vi "Latch When Pressed for Time.vi"(4 "Time (ms)":i32, 5 "Input":bool) -> (2 "Latched Output":bool)   [LabVIEW 2014]
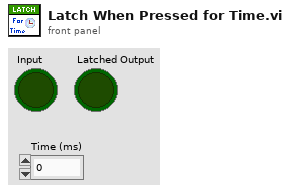
[diagram p1: front panel]
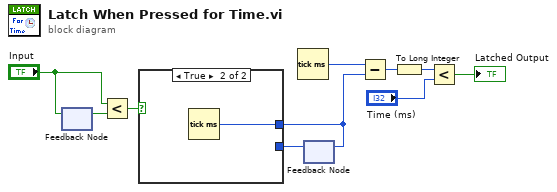
[diagram p0: block diagram]
diagram:
  n1 = feedback-in #1("Input") -> ()
  n2 = feedback #1() -> (w10:bool)  [unwired: 1 in]
  n3 = Less?(x="Input", y=w10) -> (x < y?=w8:bool)
  n4 = Tick Count (ms)() -> (millisecond timer value=w6:u32)
  n5 = feedback #2() -> (w7:u32)  [unwired: 1 in]
  n6 = case shown="True" w8 {
    tunnel: [w11 w12] -> w5
    tunnel: w7 -> [w11 _]
    frame False {
    }
    frame True {
      n7 = Tick Count (ms)() -> (millisecond timer value=w12:u32)
    }
  }
  n8 = feedback-in #2(w5) -> ()
  n9 = Subtract(x=w6, y=w5) -> (x-y=w4:u32)
  n10 = To Long Integer(number=w4) -> (32bit integer=w2:i32)
  n11 = Less?(x=w2, y="Time (ms)") -> (x < y?=→"Latched Output":bool)
